vi "Close.vi"(8 "error in (no error)":errorcluster, 11 "Host Adapter in":refnum<class "Host Adapter.lvclass">) -> (0 "error out":errorcluster, 3 "Host Adapter out":refnum<class "Host Adapter.lvclass">)   [LabVIEW 2014, in "Host Adapter.lvlib" / "Host Adapter.lvclass"]
uses:
  Host Adapter.lvclass
  Generic Instrument/Generic Instrument.lvclass
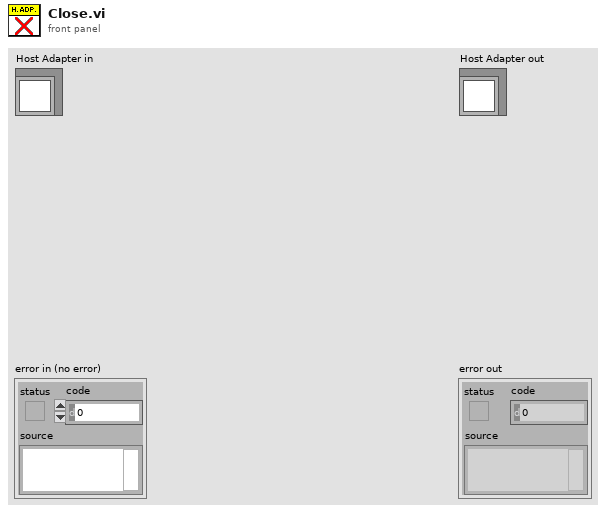
[diagram p1: front panel]
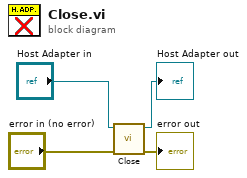
[diagram p0: block diagram]
diagram:
  n1 = call-parent "Close.vi"("error in (no error)"="error in (no error)", "Generic Instrument in"="Host Adapter in") -> ("error out"=→"error out":errorcluster, "Generic Instrument out"=→"Host Adapter out":refnum<class "Host Adapter.lvclass">)  [unwired: 8 in]
